vi "PH_Beckhoff_PP_PU.calc Ignitron State.vi"(1 "GUI Refs: Device on, heating on, water on":refnum<vi>[](array[refnum]), 2 "#: Device on, heating on, water on":i32[](array[numeric]), 3 "Digital Outputs":T2, 4 "Digital Inputs":T3, 5 "error in":errorcluster, 7 "PU Type":T1) -> (17 "Ignitron Status":T4 items=["no info", "off/false/out", "on/true/in", "Failure", "Alarm", "Status 1", "Status 2", "Status 3"], 19 "error out":errorcluster)   [LabVIEW 2014, in "PH_Beckhoff_PP_PU.lvlib"]
uses:
  PH_Beckhoff_PP_PU.lvlib
  PH_Basics/PH_StatusHandler/PH_StatusHandler.Status.ctl
  PH_Beckhoff/PH_Beckhoff.Digital Inputs.ctl
  PH_Beckhoff/PH_Beckhoff.Digital Outputs.ctl
  PH_Beckhoff_PP_PU.PU Rack Type.ctl
  PH_Basics/PH_StatusHandler/PH_StatusHandler.lvlib
  PH_Beckhoff/PH_Beckhoff.lvlib
  PH_Basics/PH_Common/PH_Common.lvlib
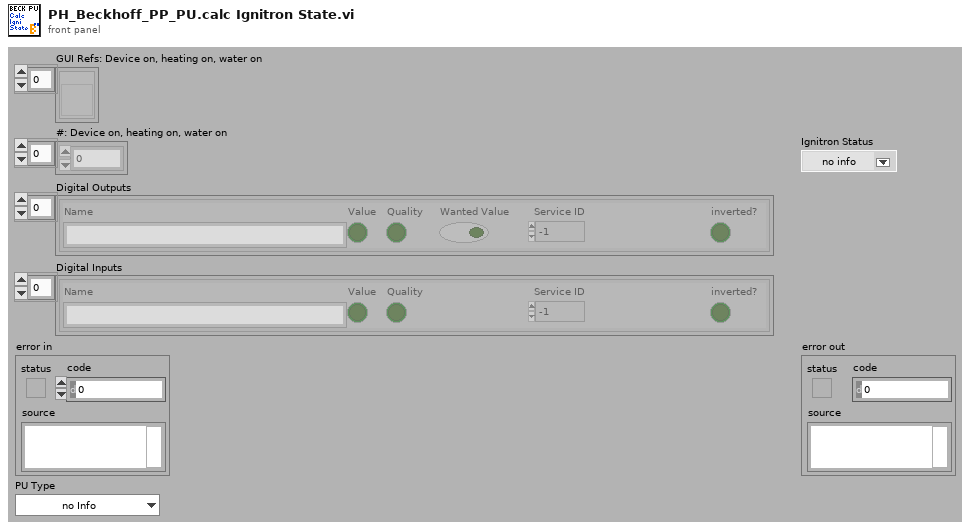
[diagram p1: front panel]
types:
  T1 = typedef "PH_Beckhoff_PP_PU.lvlib/PH_Beckhoff_PP_PU.PU Rack Type.ctl" = enum16{"no Info", "PA 19mm", "PA 45mm", "MA PU 1 and 2", "MA PU 3 and 4", "MA PU 5 and 6", "MA FR and PILC"}
  T2 = typedef "PH_Beckhoff.lvlib/PH_Beckhoff.Digital Outputs.ctl" = cluster{"Name":string, "Value":bool, "Quality":bool, "Wanted Value":bool, "Service ID":i32, "inverted?":bool}[]
  T3 = typedef "PH_Beckhoff.lvlib/PH_Beckhoff.Digital Inputs.ctl" = cluster{"Name":string, "Value":bool, "Quality":bool, "Service ID":i32, "inverted?":bool}[]
  T4 = typedef "PH_StatusHandler.lvlib/PH_StatusHandler.Status.ctl" = i16
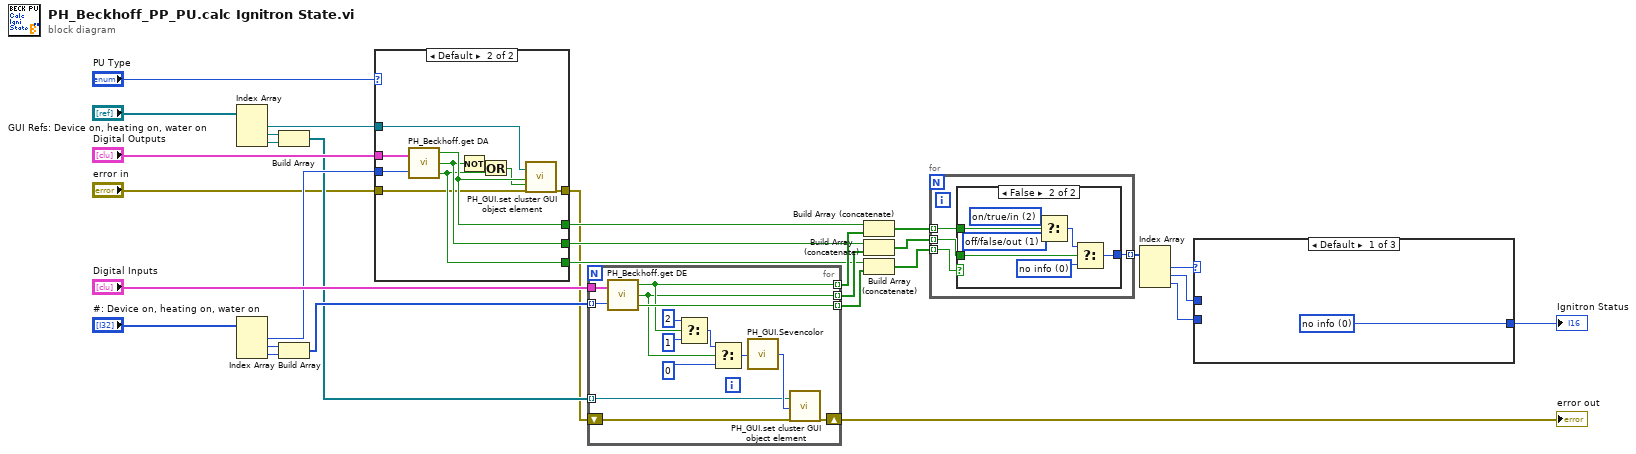
[diagram p0: block diagram]
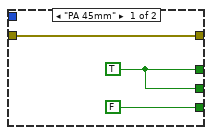
[diagram p2: hidden frame]
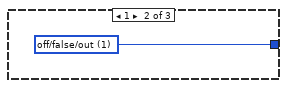
[diagram p3: hidden frame]
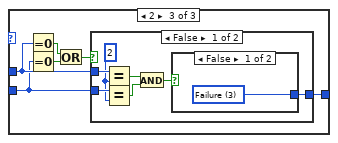
[diagram p4: hidden frame]
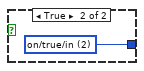
[diagram p5: hidden frame]
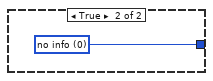
[diagram p6: hidden frame]
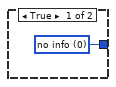
[diagram p7: hidden frame]
diagram:
  n1 = Index Array(array="GUI Refs: Device on, heating on, water on") -> (element #1=w8:refnum<vi>, element #2=w11:refnum<vi>, element #3=w10:refnum<vi>)  [unwired: 3 in]
  n2 = Index Array(array="#: Device on, heating on, water on") -> (element #1=w20:i32, element #2=w18:i32, element #3=w17:i32)  [unwired: 3 in]
  n3 = Build Array(w11, w10) -> (w9:refnum<vi>[])
  n4 = Build Array(w18, w17) -> (w16:i32[])
  n5 = case shown="Default" "PU Type" {
    tunnel: "Digital Outputs" -> [_ w43]
    tunnel: w20 -> [_ w42]
    tunnel: w8 -> [_ w41]
    tunnel: [w32 w40] -> w7
    tunnel: [w32 w39] -> w6
    tunnel: [FALSE ("Tag not found") w37] -> w5
    tunnel: "error in" -> [w33 w35]
    tunnel: [w33 w34] -> w2
    frame "PA 45mm" {
      w32 = TRUE ("Value")
    }
    frame Default {
      n6 = call "PH_Beckhoff.get DA.vi"("Digital Outputs"=w43, "index of element"=w42) -> ("Value"=w40:bool, "Quality"=w39:bool, "Tag not found"=w37:bool)
      n7 = Not(x=w39) -> (.not. x?=w38:bool)
      n8 = Or(x=w38, y=w37) -> (x .or. y?=w36:bool)
      n9 = call "PH_GUI.set cluster GUI object element.vi"("Ctl Refnum"=w41, "Value"=w40, "Blinking? (false)"=w36, "error in"=w35) -> ("error out"=w34:errorcluster)  [unwired: 15 in]
    }
  }
  n10 = for {
    tunnel: "Digital Inputs" -> [w57]
    tunnel: [w50] -> w23 mode=indexing
    tunnel: [w48] -> w22 mode=indexing
    tunnel: [w55] -> w21 mode=indexing
    tunnel: w16 -> [w56] mode=indexing
    shift-right: [w47] -> w4
    shift-left: w2 -> [w46]
    tunnel: w9 -> [w44] mode=indexing
    n11 = call "PH_Beckhoff.get DE.vi"("Digital Values"=w57, "index of element"=w56) -> ("Value"=w50:bool, "Quality"=w48:bool, "Tag not found"=w55:bool)
    n12 = Select(t=2 ("State"), s=w50, f=1 ("State")) -> (s? t:f=w51:i32)
    n13 = Select(t=w51, s=w48, f=0 ("State")) -> (s? t:f=w54:i32)
    n14 = call "PH_GUI.Sevencolor.vi"("State"=w54) -> ("Color Box"=w45:u32)
    n15 = call "PH_GUI.set cluster GUI object element.vi"("Ctl Refnum"=w44, "Value"=w45, "error in"=w46) -> ("error out"=w47:errorcluster)  [unwired: 16 in]
  }
  "error out" <- w4
  n16 = Build Array (concatenate)(w7, w23) -> (w13:bool[])
  n17 = Build Array (concatenate)(w6, w22) -> (w14:bool[])
  n18 = Build Array (concatenate)(w5, w21) -> (w15:bool[])
  n19 = for {
    tunnel: [w61] -> w27 mode=indexing
    tunnel: w15 -> [w60] mode=indexing
    tunnel: w14 -> [w59] mode=indexing
    tunnel: w13 -> [w58] mode=indexing
    n20 = case shown="False" w60 {
      tunnel: [w62 w69] -> w61
      tunnel: w59 -> [_ w64]
      tunnel: w58 -> [_ w63]
      frame True {
        w62 = T4 0 items=["no info", "off/false/out", "on/true/in", "Failure", "Alarm", "Status 1", "Status 2", "Status 3"] ("HV On State")
      }
      frame False {
        w65 = T4 1 items=["no info", "off/false/out", "on/true/in", "Failure", "Alarm", "Status 1", "Status 2", "Status 3"] ("HV On State")
        w66 = T4 2 items=["no info", "off/false/out", "on/true/in", "Failure", "Alarm", "Status 1", "Status 2", "Status 3"] ("HV On State")
        w68 = T4 0 items=["no info", "off/false/out", "on/true/in", "Failure", "Alarm", "Status 1", "Status 2", "Status 3"] ("HV On State")
        n21 = Select(t=w66, s=w63, f=w65) -> (s? t:f=w67:T4)
        n22 = Select(t=w67, s=w64, f=w68) -> (s? t:f=w69:T4)
      }
    }
  }
  n23 = Index Array(array=w27) -> (element #1=w26:T4, element #2=w25:T4, element #3=w24:T4)  [unwired: 3 in]
  n24 = case shown="Default" w26 {
    tunnel: [w70 w71 w74] -> w29
    tunnel: w25 -> [_ _ w73]
    tunnel: w24 -> [_ _ w72]
    frame Default {
      w70 = T4 0 items=["no info", "off/false/out", "on/true/in", "Failure", "Alarm", "Status 1", "Status 2", "Status 3"] ("Ignitron Status")
    }
    frame 1 {
      w71 = T4 1 items=["no info", "off/false/out", "on/true/in", "Failure", "Alarm", "Status 1", "Status 2", "Status 3"] ("Ignitron Status")
    }
    frame 2 {
      n25 = Equal To 0?(x=w73) -> (x = 0?=w77:bool)
      n26 = Equal To 0?(x=w72) -> (x = 0?=w76:bool)
      n27 = Or(x=w77, y=w76) -> (x .or. y?=w75:bool)
      n28 = case shown="False" w75 {
        tunnel: [w78 w87] -> w74
        tunnel: w73 -> [w83 _]
        tunnel: w72 -> [w84 _]
        frame False {
          w82 = 2 ("y")
          n29 = Equal?(x=w83, y=w82) -> (x = y?=w81:bool)
          n30 = Equal?(x=w84, y=w82) -> (x = y?=w80:bool)
          n31 = And(x=w81, y=w80) -> (x .and. y?=w79:bool)
          n32 = case shown="False" w79 {
            tunnel: [w85 w86] -> w78
            frame False {
              w85 = T4 3 items=["no info", "off/false/out", "on/true/in", "Failure", "Alarm", "Status 1", "Status 2", "Status 3"] ("Ignitron Status")
            }
            frame True {
              w86 = T4 2 items=["no info", "off/false/out", "on/true/in", "Failure", "Alarm", "Status 1", "Status 2", "Status 3"] ("Ignitron Status")
            }
          }
        }
        frame True {
          w87 = T4 0 items=["no info", "off/false/out", "on/true/in", "Failure", "Alarm", "Status 1", "Status 2", "Status 3"] ("Ignitron Status")
        }
      }
    }
  }
  "Ignitron Status" <- w29
